vi "get map wall.vi"(8 "error in (no error)":errorcluster, 11 "data array":string[](array[string])) -> (0 "error out":errorcluster, 3 "<JSON> wall array":string)   [LabVIEW 2019]
uses:
  <vilib>/JDP Science/JSONtext/String Subset.vi
  <vilib>/JDP Science/JSONtext/support/Strip Quotes and Unescape.vi
  <vilib>/JDP Science/JSONtext/support/Unescape JSON string.vi
  <vilib>/JDP Science/JSONtext/Parsing/Parse Full Path or Item Name.vi
  <vilib>/JDP Science/JSONtext/Offset/Find Item Locations by Path.vi
  <vilib>/JDP Science/JSONtext/JSONtext.lvlib
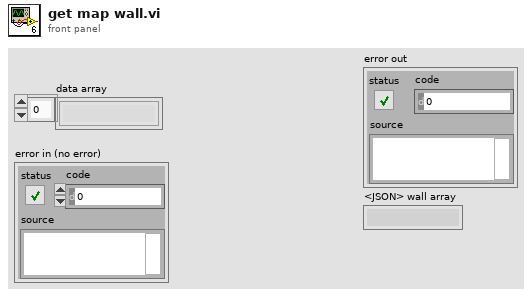
[diagram p1: front panel]
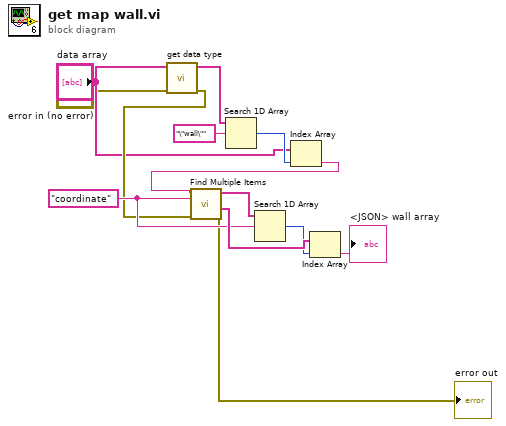
[diagram p0: block diagram]
diagram:
  w12 = "coordinate" ("$Path or Item Name")
  n1 = call "get data type.vi"("error in (no error)"="error in (no error)", "data array"="data array") -> ("error out"=w9:errorcluster, "data type"=w4:string[])  [unwired: 8 in]
  n2 = Search 1D Array(1D array=w4, element="\"wall\"") -> (index of element=w7:i32)  [unwired: 1 in]
  n3 = Index Array(array="data array", index=w7) -> (element=w8:string)
  n4 = call <vilib>:"Find Multiple Items.vi"("$Path or Item Name"=w12, "error in (no error)"=w9, "JSON"=w8) -> ("error out"=→"error out":errorcluster, "<JSON>"=w13:string[], "Item Names"=w11:string[])  [unwired: 5 in, 1 out]
  n5 = Search 1D Array(1D array=w11, element=w12) -> (index of element=w10:i32)  [unwired: 1 in]
  n6 = Index Array(array=w13, index=w10) -> (element=→"<JSON> wall array":string)
